vi "subImage_InitializeImage.vi"(8 "error in (no error)":errorcluster, 11 "Handle in":u32) -> (0 "error out":errorcluster, 3 "Handle out":u32, 4 "Image Info out":T1={"Status"="Ready", "scale bar (μm)"=inf, "Image"=array1024x1024[1048576 elements], "Histogram"={"max value"=453, "mean"=398, "min value"=349, "Histogram"={"X Values"=[349.52, 350.56, 351.6, 352.64000000000004, 353.68000000000006, 354.7200000000001, 355.7600000000001, 356.8000000000001, 357.84000000000015, 358.88000000000017, 359.9200000000002, 360.9600000000002, 362.0000000000002, 363.04000000000025, 364.08000000000027, 365.1200000000003, 366.1600000000003, 367.20000000000033, 368.24000000000035, 369.28000000000037, 370.3200000000004, 371.3600000000004, 372.40000000000043, 373.44000000000045, 374.4800000000005, 375.5200000000005, 376.5600000000005, 377.60000000000053, 378.64000000000055, 379.6800000000006, 380.7200000000006, 381.7600000000006, 382.80000000000064, 383.84000000000066, 384.8800000000007, 385.9200000000007, 386.9600000000007, 388.00000000000074, 389.04000000000076, 390.0800000000008, 391.1200000000008, 392.1600000000008, 393.20000000000084, 394.24000000000086, 395.2800000000009, 396.3200000000009, 397.3600000000009, 398.40000000000094, 399.44000000000096, 400.480000000001, 401.520000000001, 402.560000000001, 403.60000000000105, 404.64000000000107, 405.6800000000011, 406.7200000000011, 407.7600000000011, 408.80000000000115, 409.84000000000117, 410.8800000000012, 411.9200000000012, 412.96000000000123, 414.00000000000125, 415.04000000000127, 416.0800000000013, 417.1200000000013, 418.16000000000133, 419.20000000000135, 420.2400000000014, 421.2800000000014, 422.3200000000014, 423.36000000000143, 424.40000000000146, 425.4400000000015, 426.4800000000015, 427.5200000000015, 428.56000000000154, 429.60000000000156, 430.6400000000016, 431.6800000000016, 432.7200000000016, 433.76000000000164, 434.80000000000166, 435.8400000000017, 436.8800000000017, 437.9200000000017, 438.96000000000174, 440.00000000000176, 441.0400000000018, 442.0800000000018, 443.1200000000018, 444.16000000000184, 445.20000000000186, 446.2400000000019, 447.2800000000019, 448.3200000000019, 449.36000000000195, 450.40000000000197, 451.440000000002, 452.480000000002], "Histogram: h(x)"=[1, 0, 1, 0, 0, 0, 0, 1, 0, 2, 3, 0, 0, 0, 1, 1, 0, 4, 9, 8, 10, 21, 26, 28, 34, 154, 119, 176, 194, 271, 421, 601, 667, 990, 1403, 1876, 2665, 3703, 4776, 6660, 8548, 10841, 13082, 15767, 17625, 19251, 20235, 20235, 19157, 17812, 28764, 10625, 8397, 6381, 4845, 3578, 2694, 2049, 1523, 1242, 990, 763, 618, 513, 389, 301, 229, 180, 164, 124, 79, 59, 40, 39, 27, 44, 17, 16, 13, 9, 8, 6, 5, 7, 5, 2, 1, 1, 2, 1, 2, 5, 2, 1, 0, 0, 0, 3, 0, 2]}}, "Scale Info"={"Pixel size (nm)"=inf, "Total x width (μm)"=inf, "Total y width (μm)"=inf}, "Camera View indicator"=array1024x1024[1048576 elements], "max frame rate (Hz)"=200.0})   [LabVIEW 2015]
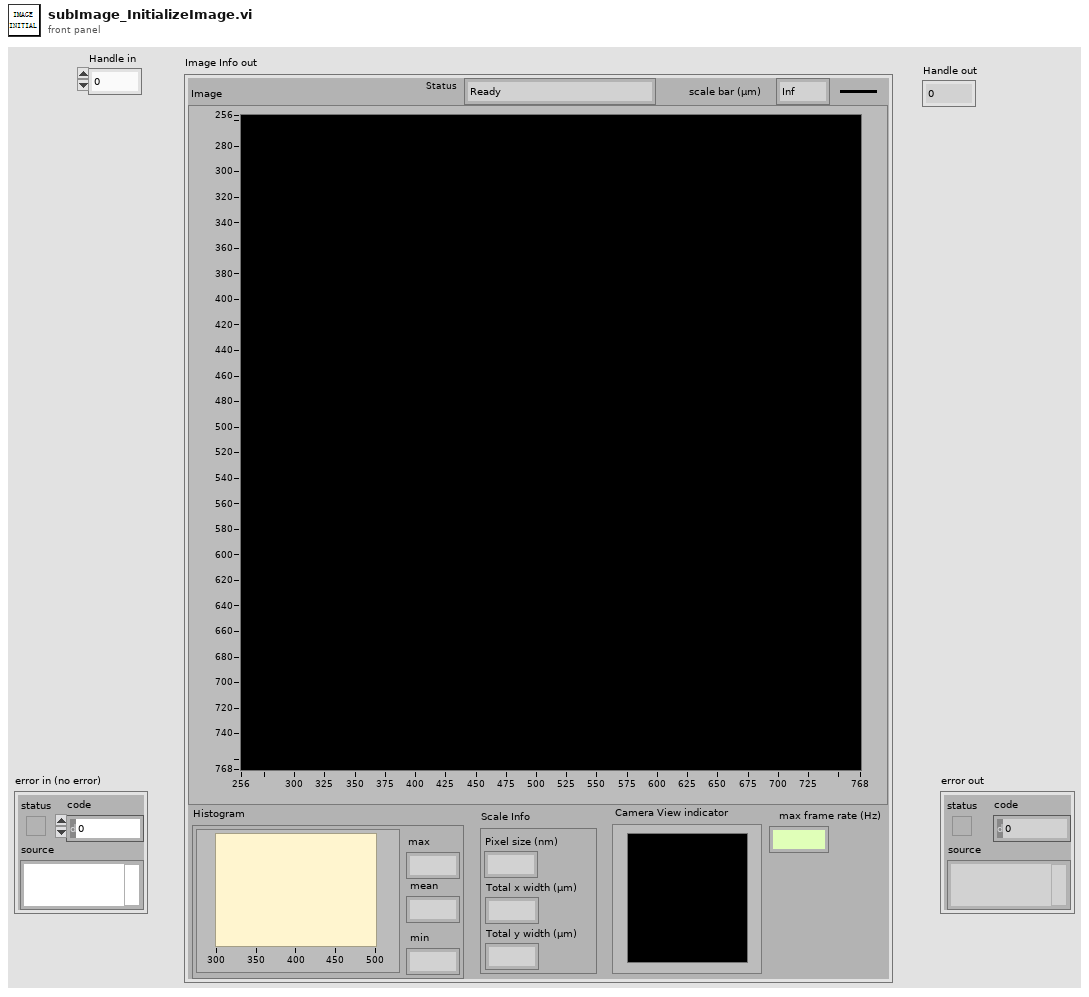
[diagram p1: front panel]
types:
  T1 = cluster{"Status":string, "scale bar (μm)":dbl, "Image":u16[][], "Histogram":cluster{"max value":u16, "mean":i16, "min value":u16, "Histogram":cluster{"X Values":dbl[], "Histogram: h(x)":i32[]}}, "Scale Info":cluster{"Pixel size (nm)":dbl, "Total x width (μm)":dbl, "Total y width (μm)":dbl}, "Camera View indicator":u16[][], "max frame rate (Hz)":dbl}
  T2 = cluster{"Value":i32, "Minimum":i32, "Maximum":i32, "Increment":i32}
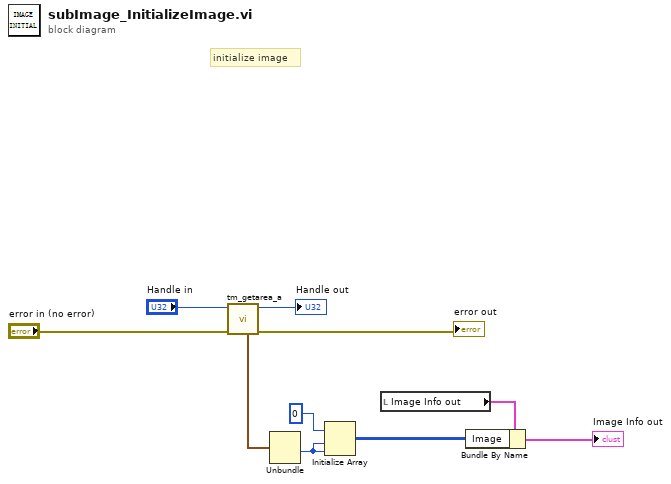
[diagram p0: block diagram]
diagram:
  # "initialize image"
  n1 = call "tm_getarea_a.vi"("error in (no error)"="error in (no error)", "Handle in"="Handle in") -> ("error out"=→"error out":errorcluster, "Handle out"=→"Handle out":u32, "H Width"=w8:T2)  [unwired: 4 in, 3 out]
  n2 = Unbundle(w8) -> ("Maximum"=w10:i32)  [unwired: 3 out]
  n3 = Initialize Array(u16 0 ("element"), w10, w10) -> (w1:u16[][])
  n4 = local read "Image Info out"() -> (w3:T1)
  n5 = Bundle By Name(cluster=w3, "Image"=w1) -> (→"Image Info out":T1)
